vi "SR_M-Mission_Util.vi"() -> ()   [LabVIEW 2015, in "Shore Library.lvlib"]
uses:
  Shore Library.lvlib
  RDS Mission Controller Actor/MissionOp.ctl
  <vilib>/Utility/miscctls.llb/LVAnnotationListTypeDef.ctl
  RDS Mission Controller Actor/RDS Mission Controller Actor.lvlib
panel:
  in  "btn_edit_op":bool
  in  "show markers":bool
  out "markers":T1
  in  "btn_load-markers":bool
  in  "Op Selektor":i16(knob) scale=0.0..1.0
  in  "btn_Turneffe":bool
  in  "btn_beach 2":bool
  in  "btn_beach1":bool
  out "Loaded Mission":T2[](array[typedef]) {"GPS Longitude" format="%.6g"; "GPS Latitude" format="%.6g"}
  in  "btn_close":bool
  in  "btn_delete_op":bool
  in  "Map Add":bool
  in  "btn_load":bool
  in  "btn_save":bool
  in  "btn_add-op":bool
  out "XY Graph":cluster{dbl[], dbl[]}(graph)
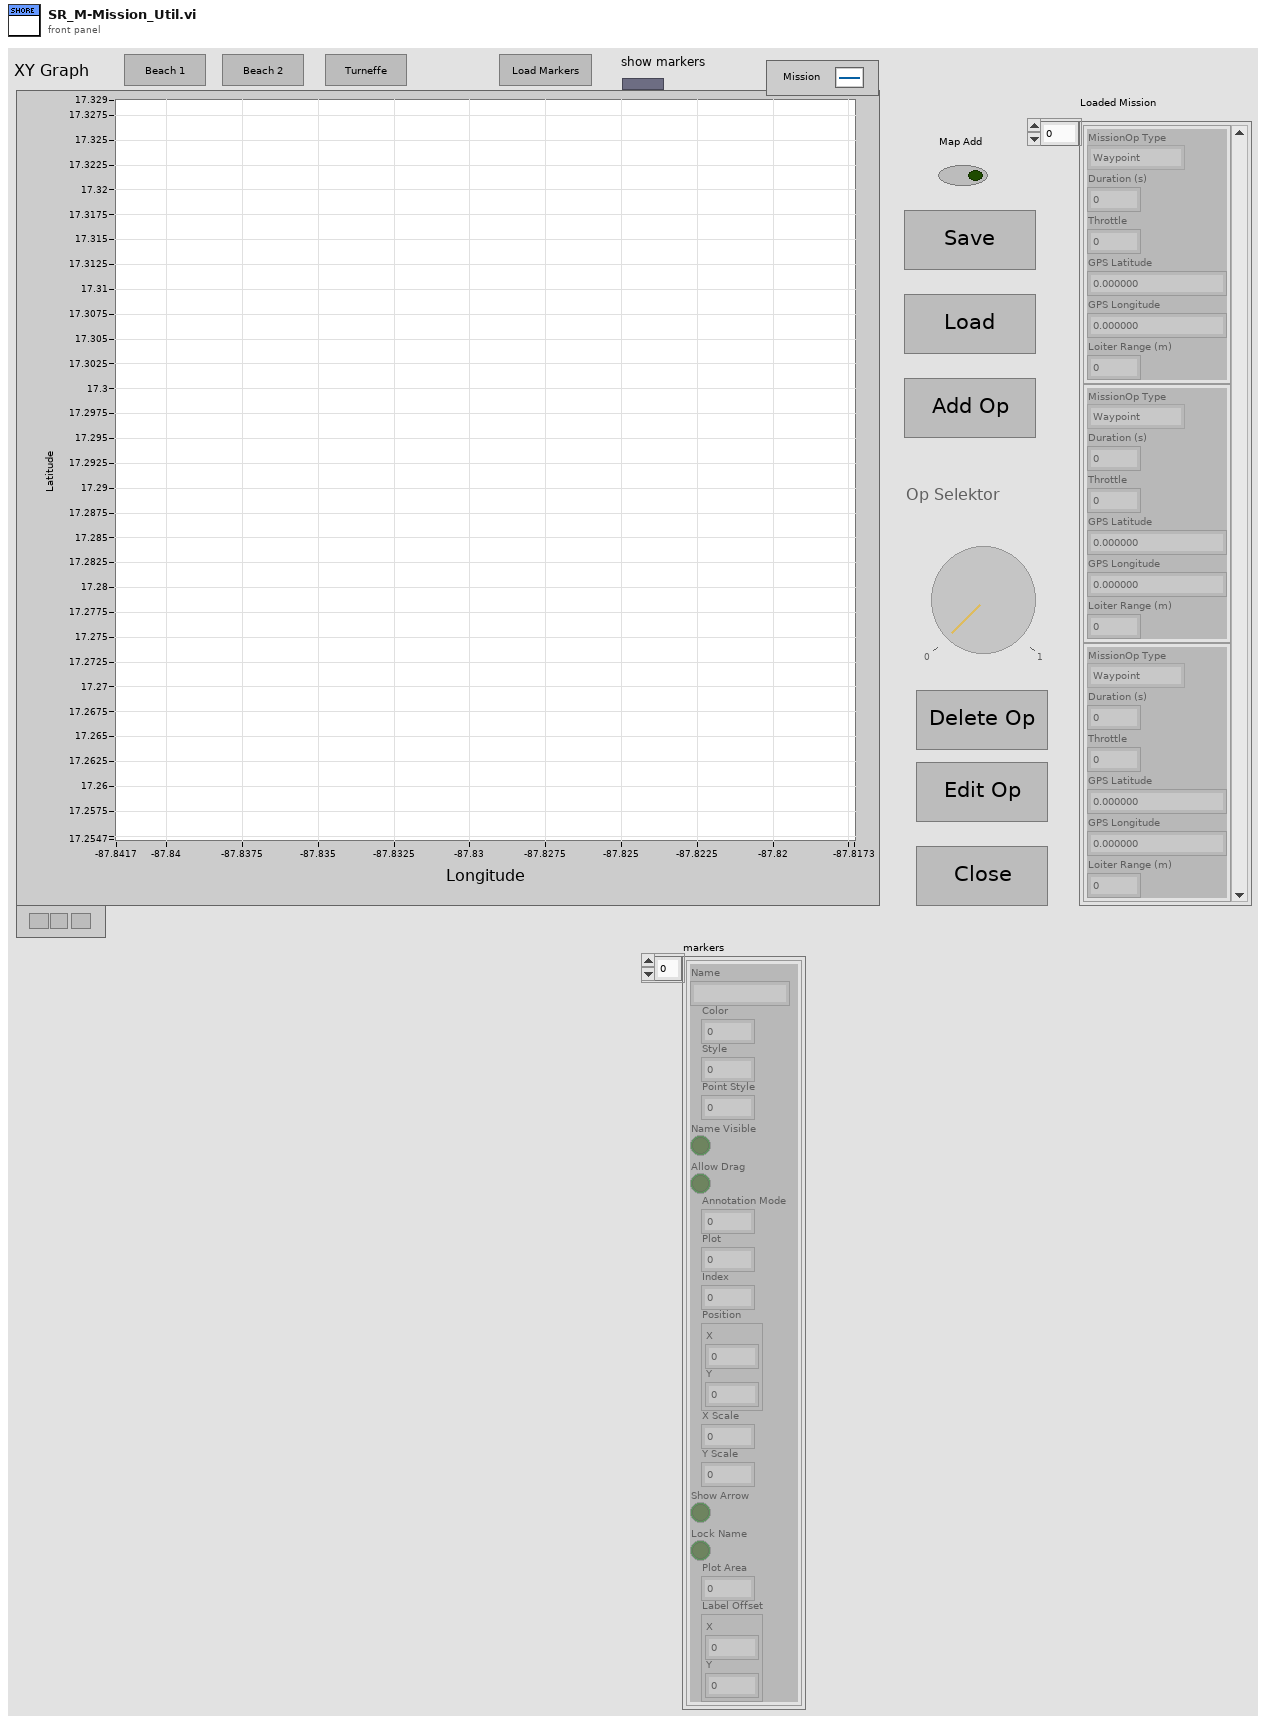
[diagram p1: front panel]
types:
  T1 = typedef "LVAnnotationListTypeDef.ctl" = cluster{"Name":string, "Color":u32, "Style":u8, "Point Style":u8, "Name Visible":bool, "Allow Drag":bool, "Annotation Mode":u32, "Plot":i32, "Index":i32, "Position":cluster{"X":dbl, "Y":dbl}, "X Scale":u32, "Y Scale":u32, "Show Arrow":bool, "Lock Name":bool, "Plot Area":i32, "Label Offset":cluster{"X":dbl, "Y":dbl}}[]
  T2 = typedef "RDS Mission Controller Actor.lvlib/MissionOp.ctl" = cluster{"MissionOp Type":enum16{"Waypoint", "Loiter", "Wait", "Deploy AIP", "Stow AIP"}, "Duration (s)":u16, "Throttle":i16, "GPS Latitude":dbl, "GPS Longitude":dbl, "Loiter Range (m)":u16}
  T3 = enum8{"Enabled", "Disabled", "Disabled and Grayed Out"}
  T4 = typedef "LVPoint32TypeDef.ctl" = cluster{"Horizontal":i32, "Vertical":i32}
  T5 = cluster{"Name":string, "Color":u32, "Style":u8, "Point Style":u8, "Name Visible":bool, "Allow Drag":bool, "Annotation Mode":u32, "Plot":i32, "Index":i32, "Position":cluster{"X":dbl, "Y":dbl}, "X Scale":u32, "Y Scale":u32, "Show Arrow":bool, "Lock Name":bool, "Plot Area":i32, "Label Offset":cluster{"X":dbl, "Y":dbl}}[]
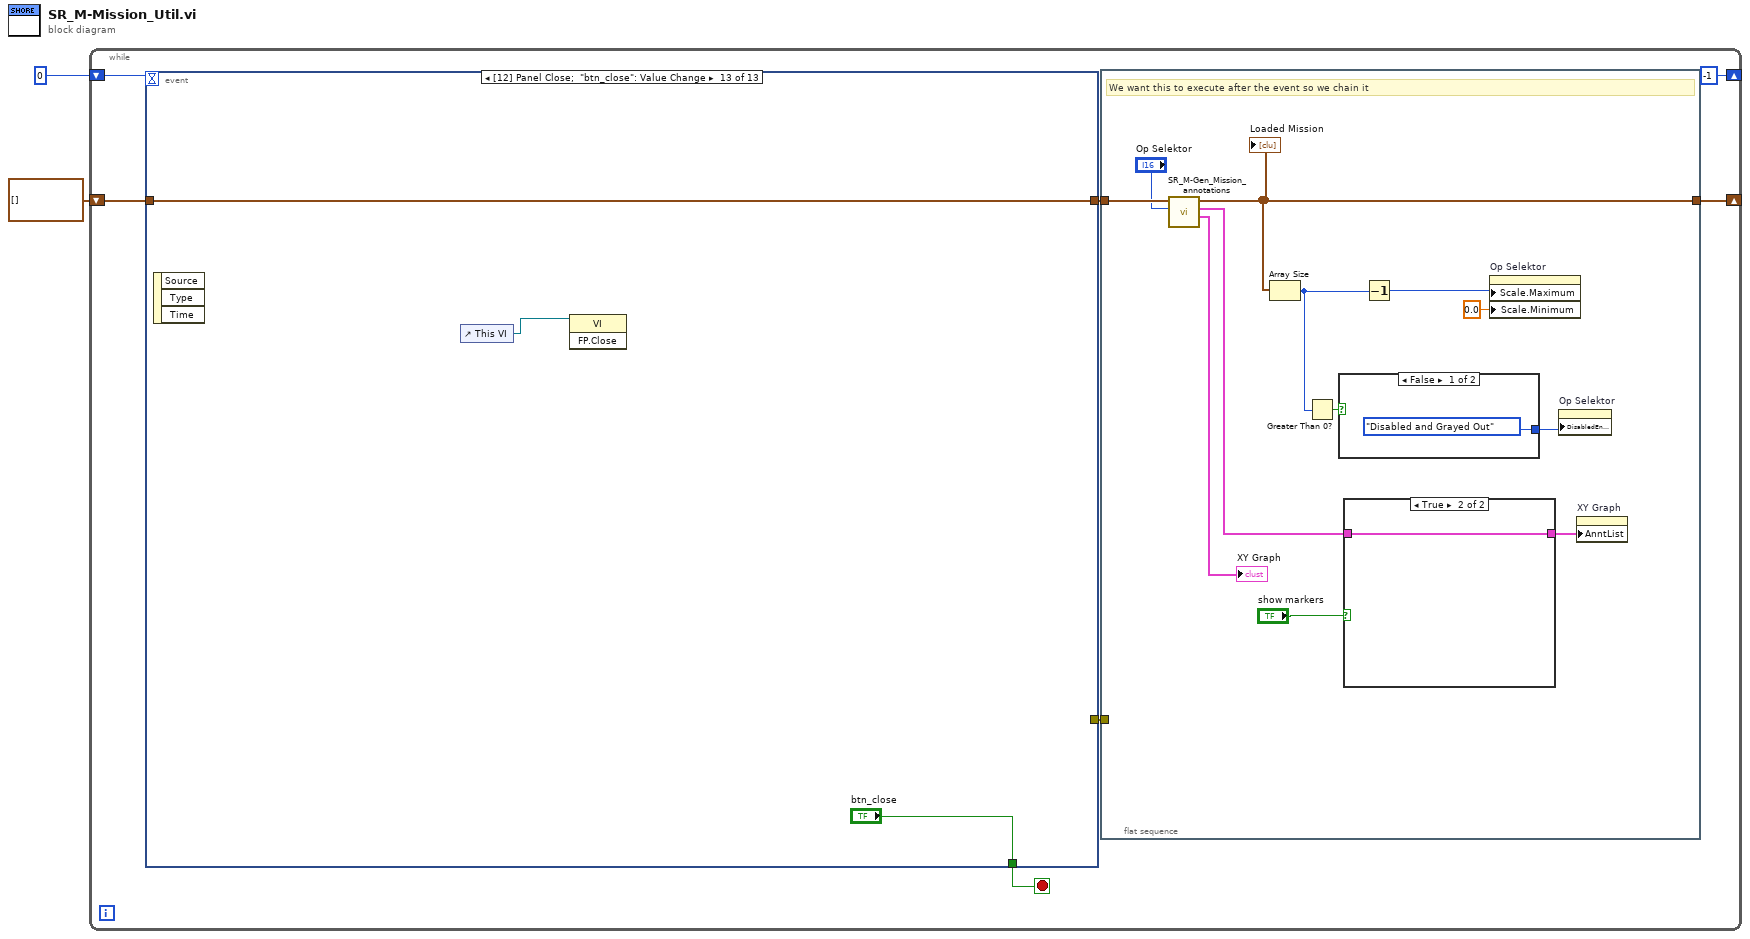
[diagram p0: block diagram]
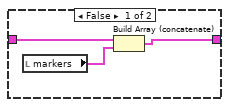
[diagram p2: hidden frame]
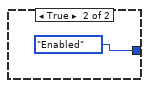
[diagram p3: hidden frame]
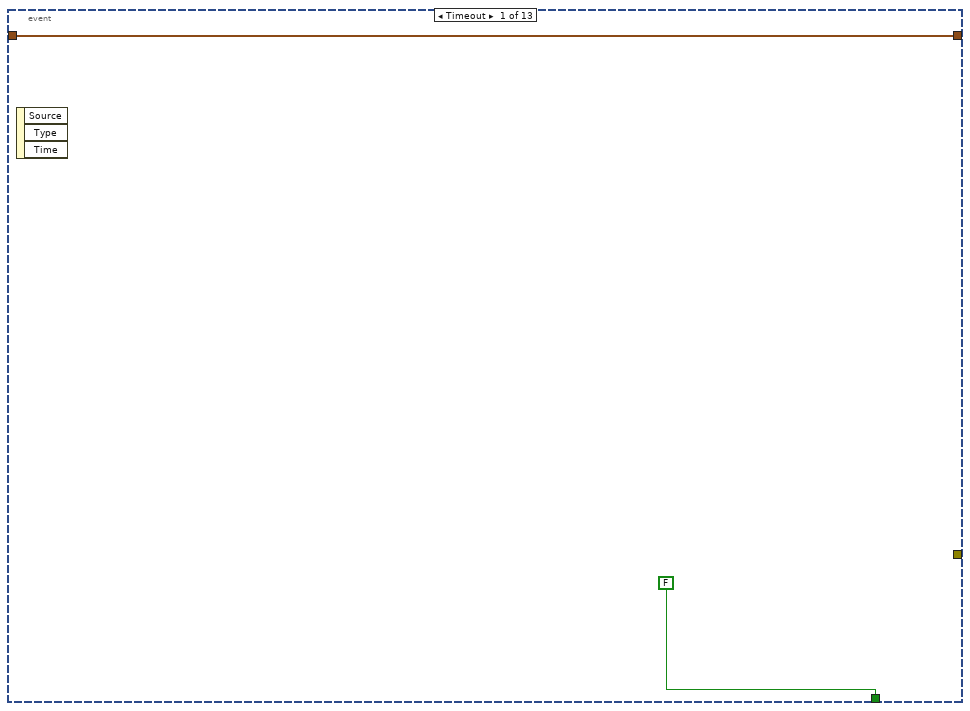
[diagram p4: hidden frame]
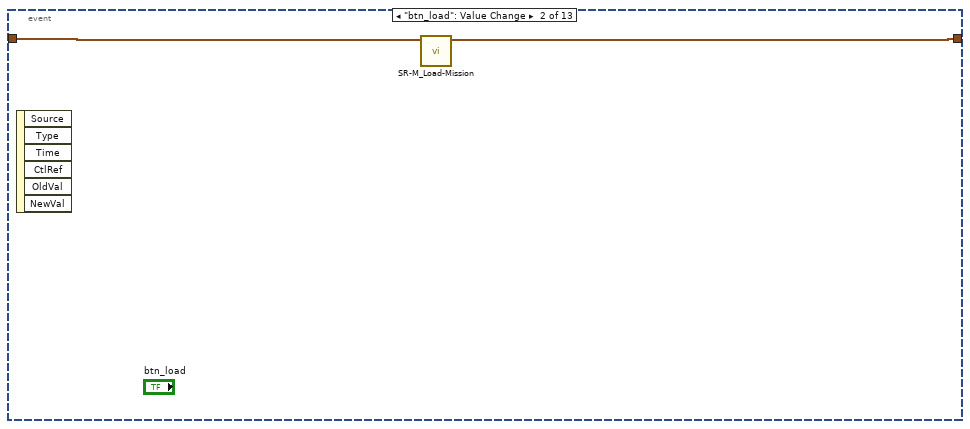
[diagram p5: hidden frame]
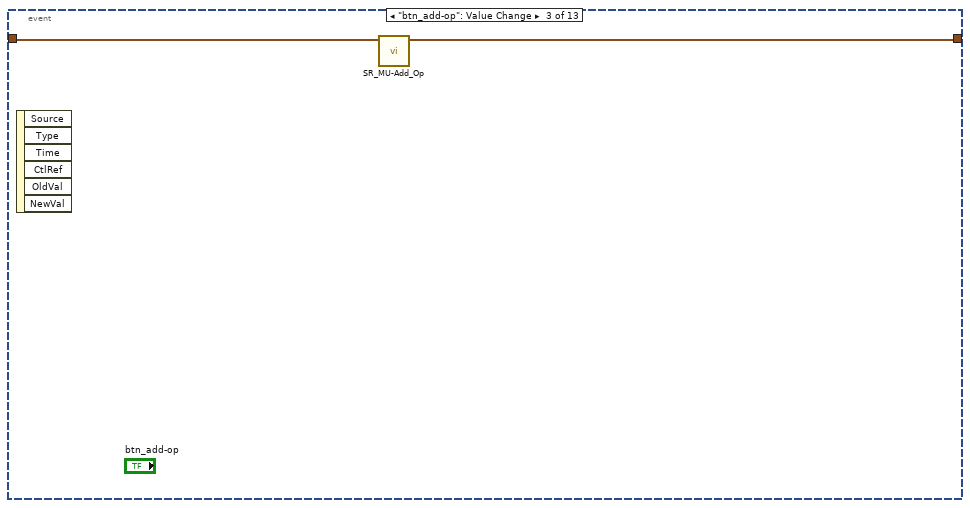
[diagram p6: hidden frame]
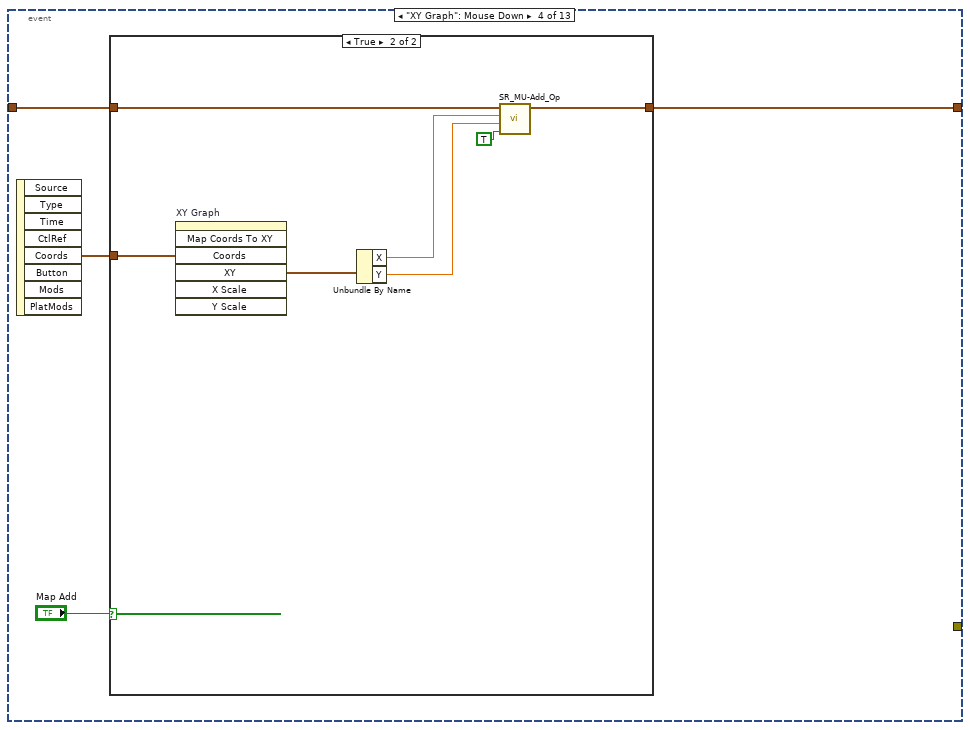
[diagram p7: hidden frame]
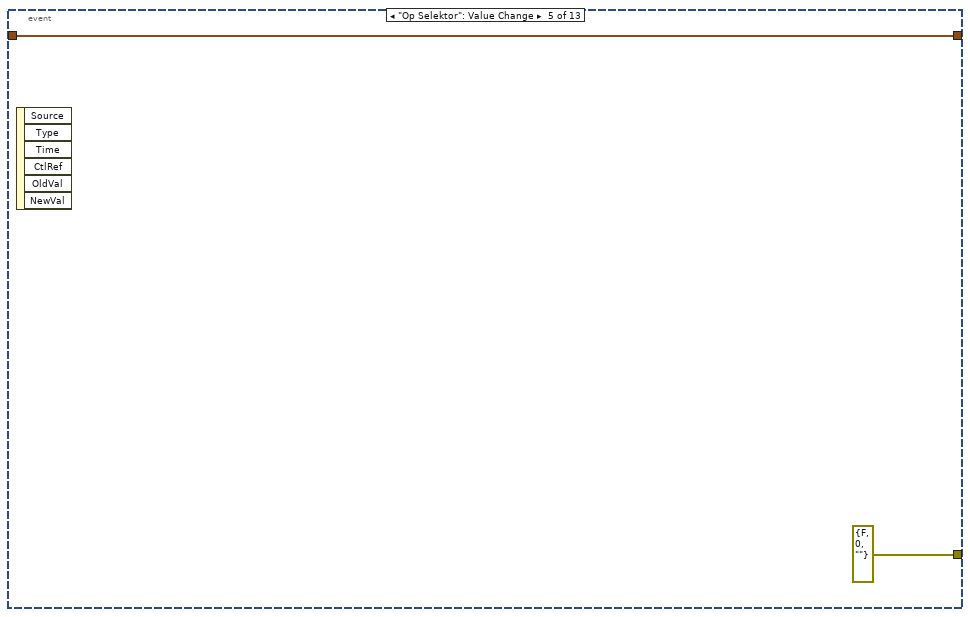
[diagram p9: hidden frame]
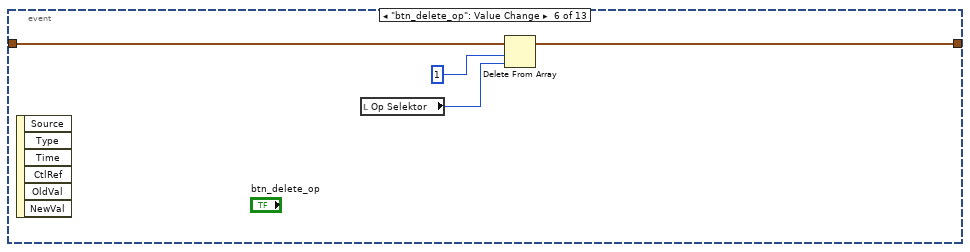
[diagram p10: hidden frame]
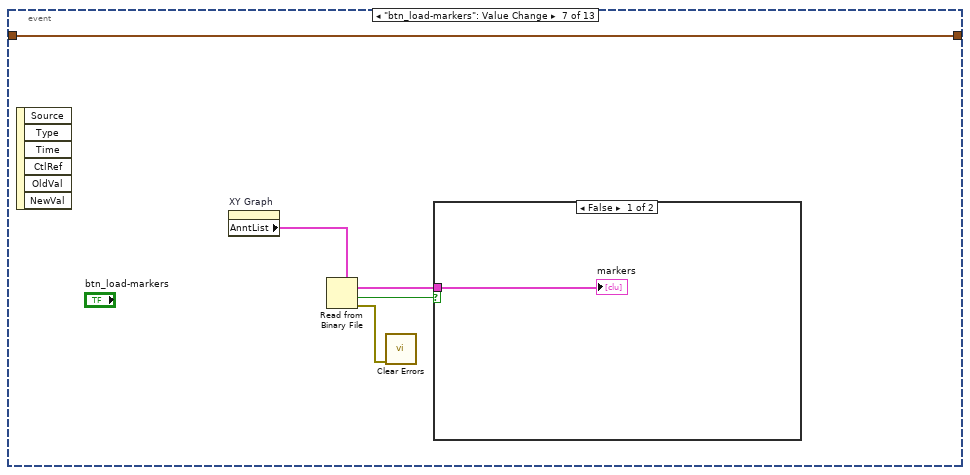
[diagram p11: hidden frame]
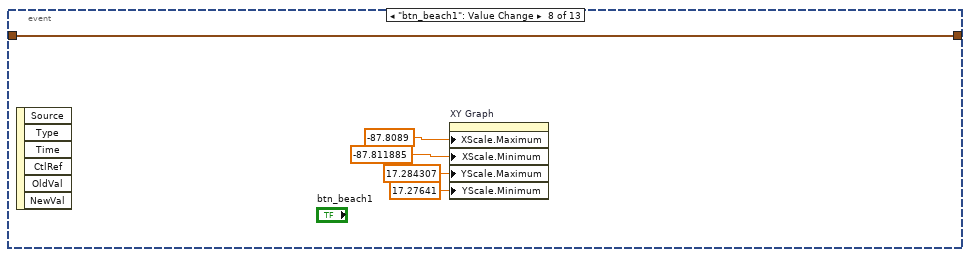
[diagram p13: hidden frame]
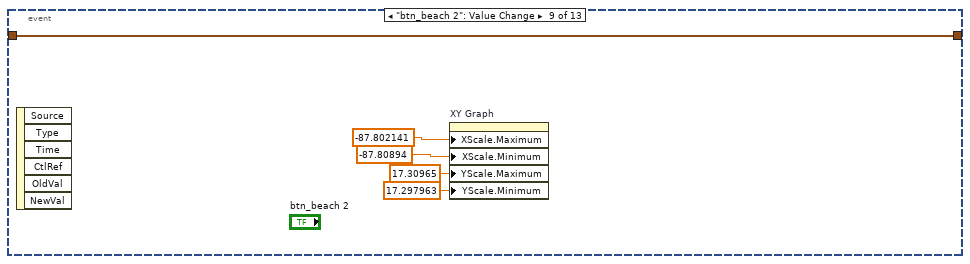
[diagram p14: hidden frame]
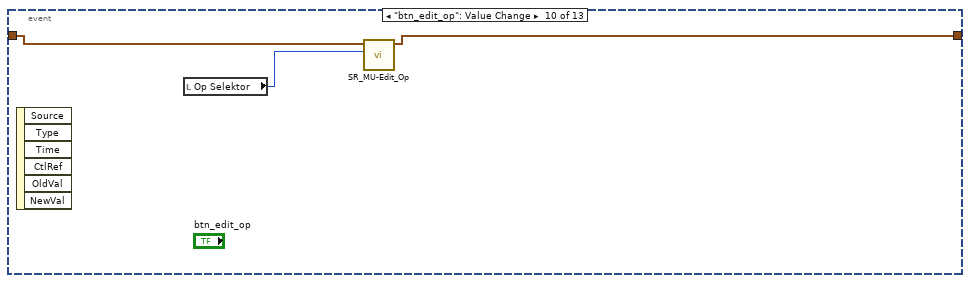
[diagram p15: hidden frame]
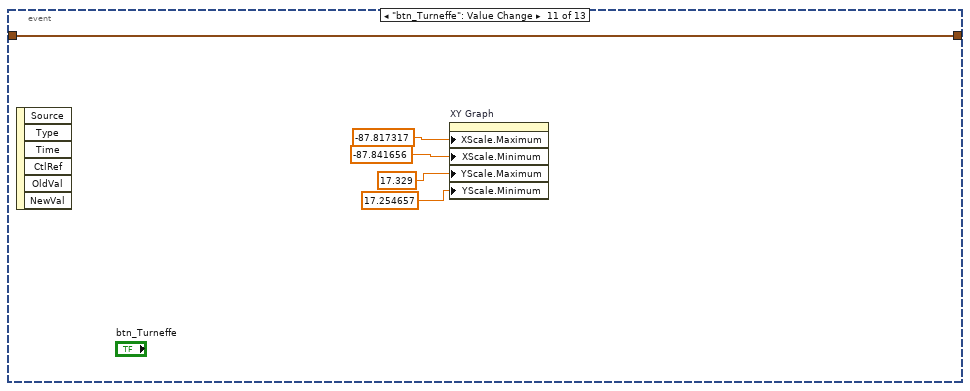
[diagram p16: hidden frame]
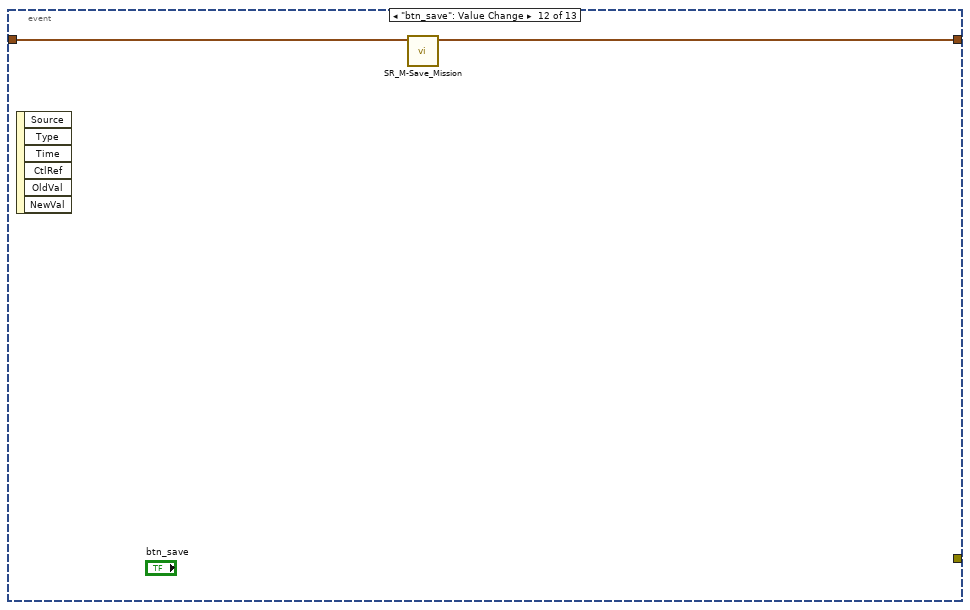
[diagram p17: hidden frame]
diagram:
  n1 = while {
    shift-right: [w6] -> _
    shift-left: T2[] [] ("Mission In") -> [w8]
    shift-right: [-1] -> _
    shift-left: 0 -> [w4]
    stop <- w9 stop-if-true
    n2 = event shown="[12] Panel Close;  \"btn_close\": Value Change" {
      selector: _ -> [_ _ _ _ _ _ _ _ _ _ _ _ _]
      dyn-events: _ -> [_ _ _ _ _ _ _ _ _ _ _ _ _]
      timeout: w4 -> [_ _ _ _ _ _ _ _ _ _ _ _ _]
      tunnel: [FALSE _ _ _ _ _ _ _ _ _ _ _ "btn_close"] -> w9
      tunnel: w8 -> [w28 w31 w33 w35 w47 w51 w56 w62 w67 w70 w75 w77 w79]
      tunnel: [w28 w30 w32 w34 w47 w50 w56 w62 w67 w68 w75 w76 w79] -> w7
      tunnel: [_ _ _ _ errorcluster {"status"=FALSE, "code"=0, "source"=""} ("error in (no error)") _ _ _ _ _ _ _ _] -> w5
      event Timeout {
        n3 = event-data() -> ()  [unwired: 1 in, 3 out]
      }
      event "btn_load": Value Change {
        n4 = event-data() -> ()  [unwired: 1 in, 6 out]
        n5 = call "SR-M_Load-Mission.vi"("Mission In in"=w31) -> ("Mission In out"=w30:T2[])  [unwired: 10 in]
      }
      event "btn_add-op": Value Change {
        n6 = event-data() -> ()  [unwired: 1 in, 6 out]
        n7 = call "SR_MU-Add_Op.vi"("Mission In"=w33) -> ("Mission Out"=w32:T2[])  [unwired: 8 in, 2 out]
      }
      event "XY Graph": Mouse Down {
        n8 = event-data() -> ("Coords"=w36:T4)  [unwired: 1 in, 7 out]
        n9 = case shown="True" "Map Add" {
          tunnel: w36 -> [_ w45]
          tunnel: w35 -> [w38 w43]
          tunnel: [w38 w39] -> w34
          frame False {
          }
          frame True {
            n10 = invoke on="XY Graph" class="XYGraph (strict)" method="Map Coords To XY"("Coords"=w45) -> ("XY"=w44:cluster{"X":dbl, "Y":dbl})  [unwired: 6 in, 6 out]
            n11 = Unbundle By Name(w44) -> ("X"=w42:dbl, "Y"=w41:dbl)
            n12 = call "SR_MU-Add_Op.vi"("Init"=TRUE, "Latitude In"=w41, "Longitude In"=w42, "Mission In"=w43) -> ("Mission Out"=w39:T2[])  [unwired: 5 in, 2 out]
          }
        }
      }
      event "Op Selektor": Value Change {
        n13 = event-data() -> ()  [unwired: 1 in, 6 out]
      }
      event "btn_delete_op": Value Change {
        n14 = event-data() -> ()  [unwired: 1 in, 6 out]
        n15 = local read "Op Selektor"() -> (w48:i16)
        n16 = Delete From Array(array=w51, length=1, index=w48) -> (array with subset deleted=w50:T2[])  [unwired: 1 out]
      }
      event "btn_load-markers": Value Change {
        n17 = event-data() -> ()  [unwired: 1 in, 6 out]
        n18 = property on="XY Graph" class="XYGraph (strict)"() -> ("AnntList"=w55:T1)  [unwired: 2 in, 2 out]
        n19 = Read from Binary File(5:w55) -> (0:w52:errorcluster, 1:w53:bool, 2:w54:T1)  [unwired: 5 in, 1 out]
        n20 = call <vilib>:"Clear Errors.vi"("error in (no error)"=w52) -> ()  [unwired: 5 in, 2 out]
        n21 = case shown="False" w53 {
          tunnel: w54 -> [w57 _]
          frame False {
            "markers" <- w57
          }
          frame True {
          }
        }
      }
      event "btn_beach1": Value Change {
        n22 = event-data() -> ()  [unwired: 1 in, 6 out]
        n23 = property on="XY Graph" class="XYGraph (strict)"("XScale.Maximum"=-87.8089 ("X Scale.Range:Maximum"), "XScale.Minimum"=-87.811885 ("X Scale.Range:Maximum"), "YScale.Maximum"=17.284307 ("X Scale.Range:Maximum"), "YScale.Minimum"=17.27641 ("X Scale.Range:Maximum")) -> ()  [unwired: 2 in, 2 out]
      }
      event "btn_beach 2": Value Change {
        n24 = event-data() -> ()  [unwired: 1 in, 6 out]
        n25 = property on="XY Graph" class="XYGraph (strict)"("XScale.Maximum"=-87.802141 ("X Scale.Range:Maximum"), "XScale.Minimum"=-87.80894 ("X Scale.Range:Maximum"), "YScale.Maximum"=17.30965 ("X Scale.Range:Maximum"), "YScale.Minimum"=17.297963 ("X Scale.Range:Maximum")) -> ()  [unwired: 2 in, 2 out]
      }
      event "btn_edit_op": Value Change {
        n26 = event-data() -> ()  [unwired: 1 in, 6 out]
        n27 = local read "Op Selektor"() -> (w69:i16)
        n28 = call "SR_MU-Edit_Op.vi"("Index"=w69, "Mission In"=w70) -> ("Mission Out"=w68:T2[])  [unwired: 7 in, 2 out]
      }
      event "btn_Turneffe": Value Change {
        n29 = event-data() -> ()  [unwired: 1 in, 6 out]
        n30 = property on="XY Graph" class="XYGraph (strict)"("XScale.Maximum"=-87.817317 ("X Scale.Range:Maximum"), "XScale.Minimum"=-87.841656 ("X Scale.Range:Maximum"), "YScale.Maximum"=17.329 ("X Scale.Range:Maximum"), "YScale.Minimum"=17.254657 ("X Scale.Range:Maximum")) -> ()  [unwired: 2 in, 2 out]
      }
      event "btn_save": Value Change {
        n31 = event-data() -> ()  [unwired: 1 in, 6 out]
        n32 = call "SR_M-Save_Mission.vi"("Mission In in"=w77) -> ("Mission In out"=w76:T2[])  [unwired: 10 in]
      }
      event Panel Close; "btn_close": Value Change {
        n33 = event-data() -> ()  [unwired: 1 in, 3 out]
        n34 = control-ref of="This VI"() -> (w78:refnum<vi>)
        n35 = invoke class="VI" method="FP.Close"(reference=w78) -> ()  [unwired: 2 in, 3 out]
      }
    }
    n36 = flat-sequence {
      tunnel: w7 -> [w21]
      tunnel: [w19] -> w6
      tunnel: w5 -> [_]
      frame #0 {
        # "We want this to execute after the event so we chain it"
        n37 = call "SR_M-Gen_Mission_annotations.vi"("Op Index"="Op Selektor", "Mission In"=w21) -> ("Mission Path"=→"XY Graph":cluster{dbl[], dbl[]}, "Mission Annotation"=w11:T5, "Mission Out"=w19:T2[])  [unwired: 7 in]
        "Loaded Mission" <- w19
        n38 = Array Size(array=w19) -> (size(s)=w14:i32)
        n39 = Greater Than 0?(x=w14) -> (x > 0?=w18:bool)
        n40 = case shown="False" w18 {
          tunnel: [T3."Disabled and Grayed Out" ("Disabled") T3."Enabled" ("Disabled")] -> w17
          frame False {
          }
          frame True {
          }
        }
        n41 = case shown="True" "show markers" {
          tunnel: [w23 w25] -> w12
          tunnel: w11 -> [w24 w25]
          frame False {
            n42 = local read "markers"() -> (w22:T1)
            n43 = Build Array (concatenate)(w24, w22) -> (w23:T1)
          }
          frame True {
          }
        }
        n44 = Decrement(x=w14) -> (x-1=w13:i32)
        n45 = property on="Op Selektor" class="Knob (strict)"("Scale.Maximum"=w13, "Scale.Minimum"=0.0 ("Scale.Range:Minimum")) -> ()  [unwired: 2 in, 2 out]
        n46 = property on="Op Selektor" class="Knob (strict)"("DisabledEnum"=w17) -> ()  [unwired: 2 in, 2 out]
        n47 = property on="XY Graph" class="XYGraph (strict)"("AnntList"=w12) -> ()  [unwired: 2 in, 2 out]
      }
    }
  }
